vi "Rate Limiter (DBL Array).vi"(2 "initialize":bool, 3 "dt":dbl format="%.6f", 4 "slew rate limit":T1 {"falling slew rate" format="%.2f"; "rising slew rate" format="%.2f"}, 5 "Input Points":dbl[](array[numeric]) format="%.2f") -> (1 "Output Points":dbl[](array[numeric]) format="%.2f")   [LabVIEW 2020, in "NI_AdvCtrl_nonlinear.lvlib"]
doc: "LabVIEW no longer supports this VI. You can obtain similar functionality by installing the LabVIEW Simulation Module.\n\nLimits the rate of change of a given signal."
uses:
  <vilib>/addons/control/advanced/NI_AdvCtrl_nonlinear.lvlib
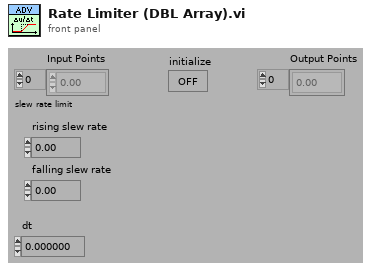
[diagram p1: front panel]
types:
  T1 = cluster{"rising slew rate":dbl, "falling slew rate":dbl}
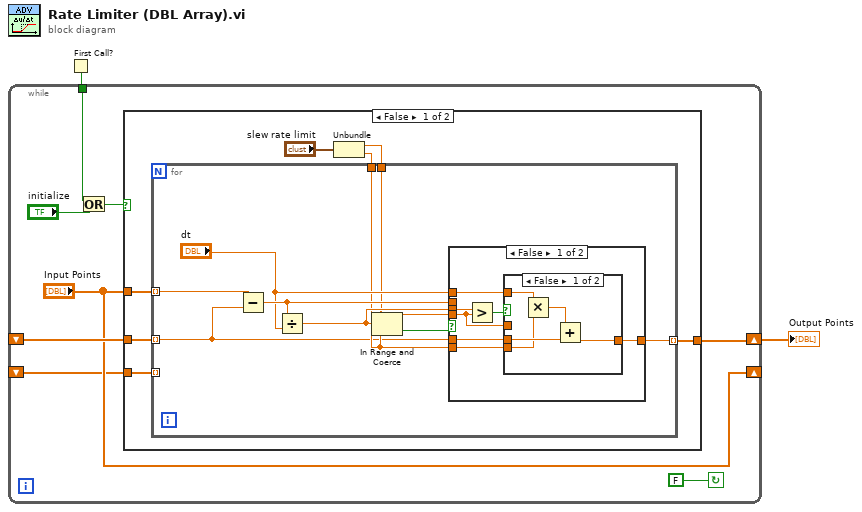
[diagram p0: block diagram]
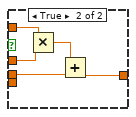
[diagram p2: hidden frame]
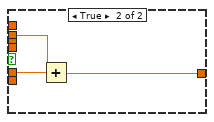
[diagram p3: hidden frame]
diagram:
  n1 = First Call?() -> (First Call?: T/F=w2:bool)
  n2 = while {
    shift-left: _ -> [w3]
    shift-right: ["Input Points"] -> _
    tunnel: w2 -> [w7]
    shift-left: _ -> [w5]
    shift-right: [w10] -> w1
    stop <- FALSE continue-if-true
    n3 = Or(x=w7, y="initialize") -> (x .or. y?=w6:bool)
    n4 = case shown="False" w6 {
      tunnel: [w17 w47] -> w10
      tunnel: "Input Points" -> [w16 w47]
      tunnel: w5 -> [w12 _]
      tunnel: w3 -> [w11 _]
      frame False {
        n5 = Unbundle("slew rate limit") -> ("rising slew rate"=w14:dbl, "falling slew rate"=w13:dbl)
        n6 = for {
          tunnel: w12 -> [w18] mode=indexing
          tunnel: [w24] -> w17 mode=indexing
          tunnel: w16 -> [w21] mode=indexing
          tunnel: w14 -> [w20]
          tunnel: w13 -> [w19]
          tunnel: w11 -> [_] mode=indexing
          n7 = Subtract(x=w21, y=w18) -> (x-y=w25:dbl)
          n8 = Divide(x=w25, y="dt") -> (x/y=w23:dbl)
          n9 = In Range and Coerce(upper limit=w20, x=w23, lower limit=w19) -> (In Range?=w26:bool)  [unwired: 1 out]
          n10 = case shown="False" w26 {
            tunnel: w25 -> [_ w46]
            tunnel: w18 -> [w29 w45]
            tunnel: [w28 w44] -> w24
            tunnel: w23 -> [w33 _]
            tunnel: w20 -> [w30 _]
            tunnel: "dt" -> [w31 _]
            tunnel: w19 -> [w27 _]
            frame False {
              n11 = Greater?(x=w33, y=w30) -> (0:w32:bool)
              n12 = case shown="False" w32 {
                tunnel: w31 -> [w38 w43]
                tunnel: w30 -> [_ w42]
                tunnel: w29 -> [w36 w40]
                tunnel: [w35 w39] -> w28
                tunnel: w27 -> [w34 _]
                frame False {
                  n13 = Multiply(x=w38, y=w34) -> (x*y=w37:dbl)
                  n14 = Add(x=w37, y=w36) -> (x+y=w35:dbl)
                }
                frame True {
                  n15 = Multiply(x=w43, y=w42) -> (x*y=w41:dbl)
                  n16 = Add(x=w41, y=w40) -> (x+y=w39:dbl)
                }
              }
            }
            frame True {
              n17 = Add(x=w46, y=w45) -> (x+y=w44:dbl)
            }
          }
        }
      }
      frame True {
      }
    }
  }
  "Output Points" <- w1
